vi "RSZVB Set Ripple Limit Range.vi"(7 "Limit (0.0)":dbl format="%^.3e", 8 "error in (no error)":errorcluster {"code" format="%.0x"}, 9 "Segment (1)":i32=1, 10 "Channel (Trace) (1)":i32=1, 11 "VISA session":refnum<visa-resource-name>) -> (0 "error out":errorcluster {"code" format="%.0x"}, 3 "dup VISA session":refnum<visa-resource-name>)   [LabVIEW 2011]
doc: "This VI defines the ripple limit for ripple limit range no. <Seg>. \n\nNotes:\n\n(1) A range must be created first to enable this command (e.g CALCulate<Chn>:RIPPle:DATA). \n\nRemote-control command(s):\nCALCulate<Chn>:RIPPle:SEGMent<Seg>:LIMit"
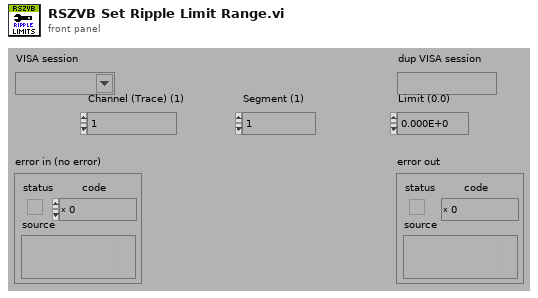
[diagram p1: front panel]
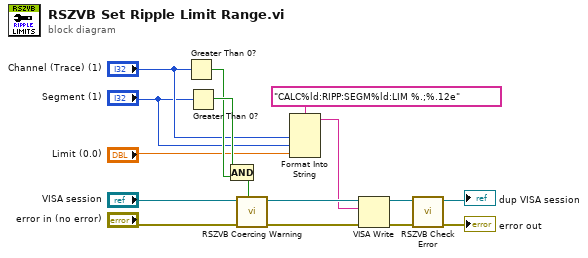
[diagram p0: block diagram]
diagram:
  n1 = Greater Than 0?(x="Channel (Trace) (1)") -> (x > 0?=w10:bool)
  n2 = Greater Than 0?(x="Segment (1)") -> (x > 0?=w11:bool)
  n3 = Compound Arithmetic op=AND(w11, w10) -> (w12:bool)
  n4 = call "RSZVB Coercing Warning.vi"("In Range?"=w12, "error in (no error)"="error in (no error)", "VISA session"="VISA session") -> ("error out"=w15:errorcluster, "dup VISA session"=w16:refnum<visa-resource-name>)  [unwired: 7 in]
  n5 = Format Into String(format string="CALC%ld:RIPP:SEGM%ld:LIM %.;%.12e", "Channel (Trace) (1)", "Segment (1)", "Limit (0.0)") -> (resulting string=w8:string)  [unwired: 2 in, 1 out]
  n6 = VISA Write(VISA resource name=w16, write buffer=w8, error in (no error)=w15) -> (VISA resource name out=w13:refnum<visa-resource-name>, error out=w14:errorcluster)  [unwired: 1 out]
  n7 = call "RSZVB Check Error.vi"("error in (no error)"=w14, "VISA session"=w13) -> ("error out"=→"error out":errorcluster, "dup VISA session"=→"dup VISA session":refnum<visa-resource-name>)  [unwired: 8 in]
